vi "InfoRead4.vi"(4 "data info template":refnum<vi>, 5 "source path":string) -> (2 "data from *.info.txt":T1)   [LabVIEW 2014]
uses:
  <vilib>/Utility/file.llb/Read From Spreadsheet File (string).vi
panel:
  # "0 - aplly *.info.txt\n1 - Continue and enter the data manually\n2 - Cancel and correct the *.info.txt"
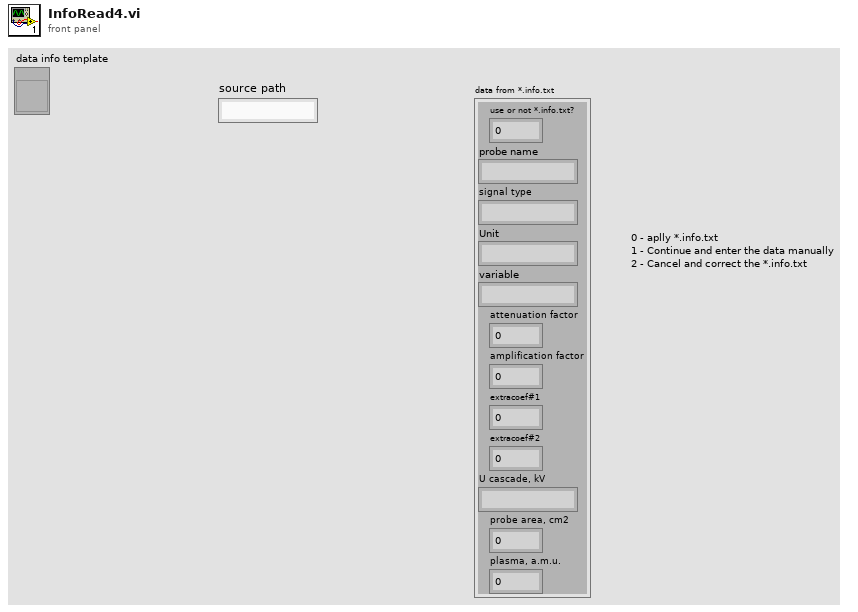
[diagram p1: front panel]
types:
  T1 = cluster{"use or not *.info.txt?":i16, "probe name":string, "signal type":string, "Unit":string, "variable":string, "attenuation factor":dbl, "amplification factor":dbl, "extracoef#1":dbl, "extracoef#2":dbl, "U cascade, kV":string, "probe area, cm2":dbl, "plasma, a.m.u.":dbl}
  T2 = cluster{"data path":string, "ADCintercadr_s":dbl, "data info":cluster{"use or not *.info.txt?":i16, "probe name":string, "signal type":string, "Unit":string, "variable":string, "attenuation factor":dbl, "amplification factor":dbl, "extracoef#1":dbl, "extracoef#2":dbl, "U cascade, kV":string, "probe area, cm2":dbl, "plasma, a.m.u.":dbl}, "channel_name":string, "channels_in_file":i32}
  T3 = enum16{"Left Button", "Center Button", "Right Button", "Window Close"}
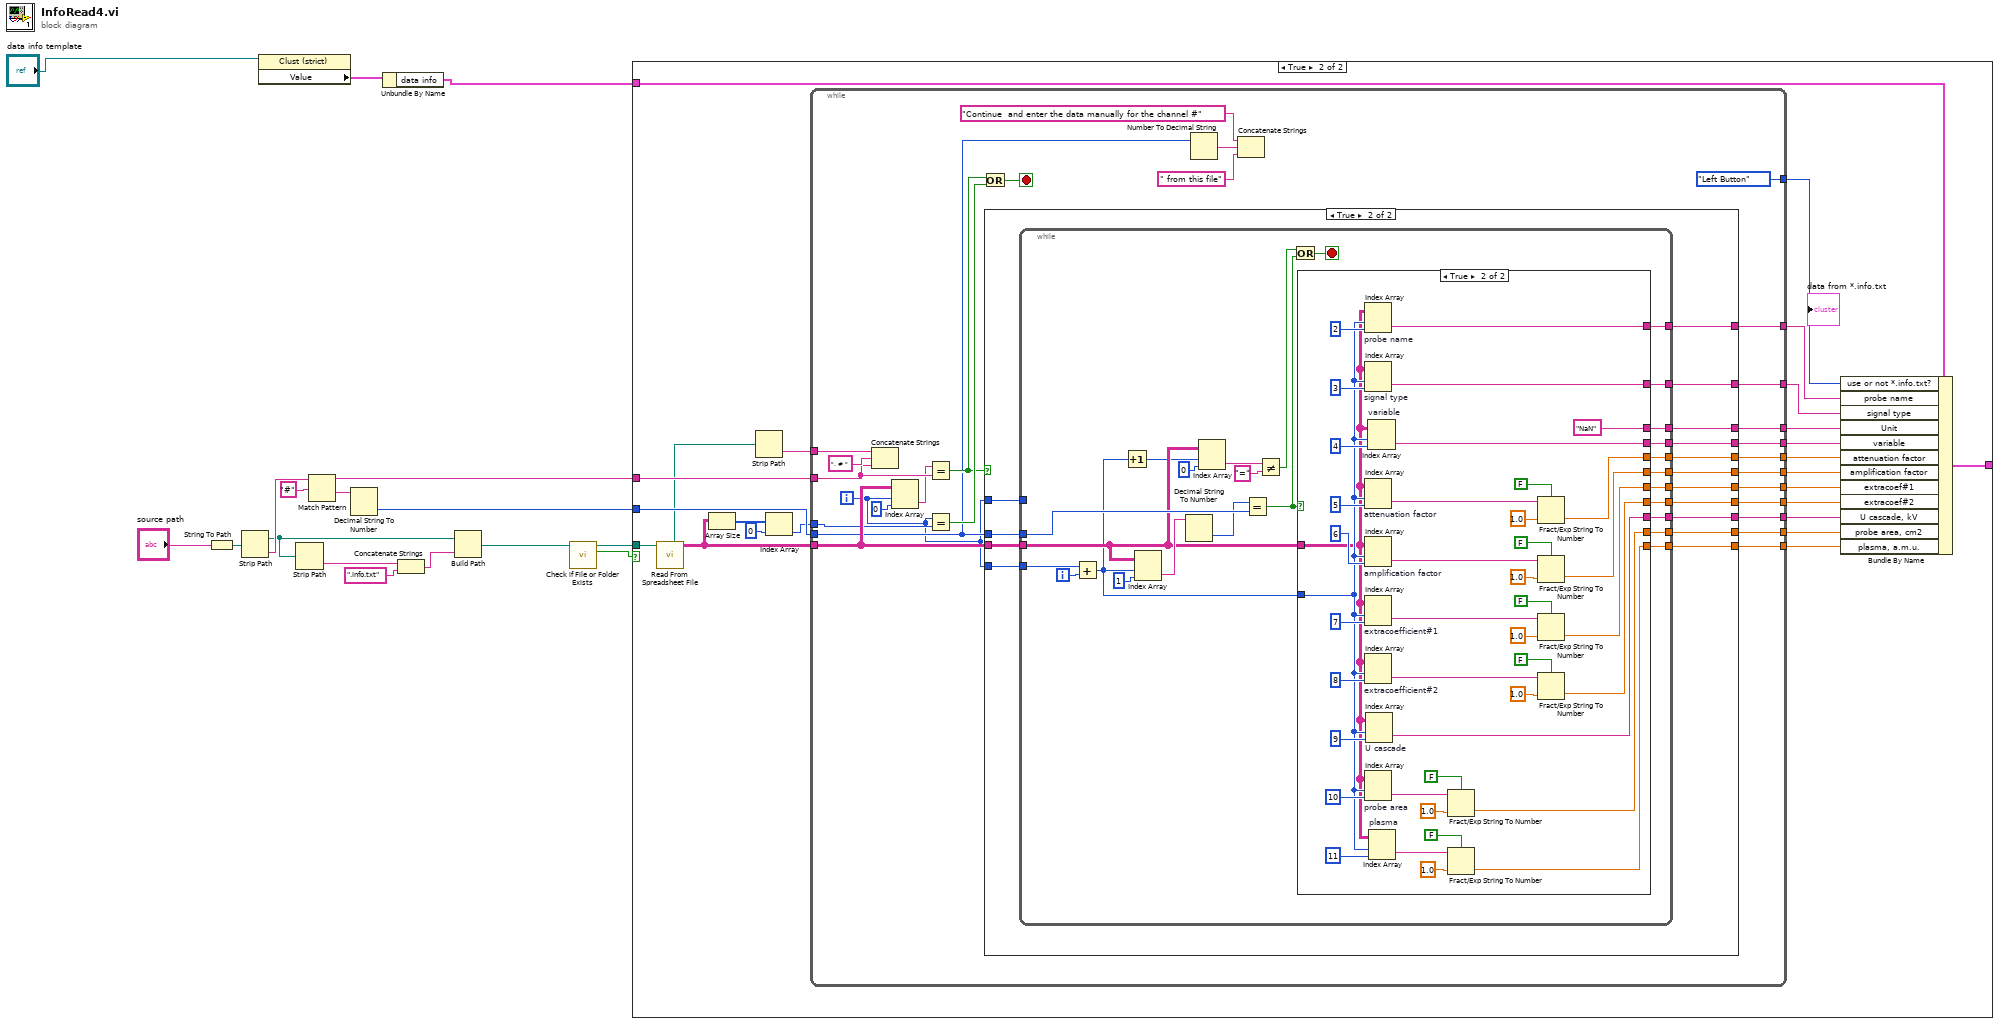
[diagram p0: block diagram]
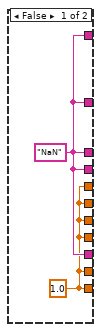
[diagram p3: hidden frame]
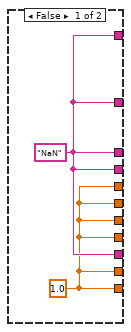
[diagram p4: hidden frame]
diagram:
  n1 = String To Path(string="source path") -> (path=w12:path)
  n2 = Strip Path(path=w12) -> (stripped path=w6:path, name=w16:string)
  n3 = property class="Clust (strict)"(reference="data info template") -> ("Value"=w3:T2)  [unwired: 1 in, 2 out]
  n4 = Strip Path(path=w6) -> (name=w5:string)  [unwired: 1 out]
  n5 = Match Pattern(string=w16, regular expression="#") -> (before substring=w11:string, after substring=w14:string)  [unwired: 1 in, 2 out]
  n6 = Decimal String To Number(string=w14) -> (number=w13:i32)  [unwired: 2 in, 1 out]
  n7 = Unbundle By Name(w3) -> ("data info"=w2:T1)
  n8 = Concatenate Strings(w5, ".info.txt" ("string")) -> (w9:string)
  n9 = Build Path(base path=w6, name or relative path=w9) -> (appended path=w8:path)
  n10 = call <vilib>:"Check if File or Folder Exists.vi"("path"=w8) -> ("file or folder exists?"=w4:bool, "dup path"=w7:path)  [unwired: 8 in, 1 out]
  n11 = case shown="True" w4 {
    tunnel: w13 -> [_ w38]
    tunnel: w11 -> [_ w37]
    tunnel: w7 -> [_ w35]
    tunnel: [w18 w19] -> _
    tunnel: w2 -> [w18 w20]
    frame False {
    }
    frame True {
      n12 = call-poly <vilib>:"Read From Spreadsheet File.vi"("file path (dialog if empty)"=w35) -> ("all rows"=w36:string[][], "new file path (Not A Path if cancelled)"=w34:path)  [unwired: 6 in, 3 out]
      n13 = Array Size(array=w36) -> (size(s)=w40:i32[])
      n14 = Strip Path(path=w34) -> (name=w39:string)  [unwired: 1 out]
      n15 = Index Array(array=w40, index=0) -> (element=w33:i32)
      n16 = while {
        tunnel: w36 -> [w64]
        tunnel: [T3."Left Button" ("Which Button?")] -> w32
        tunnel: w38 -> [w58]
        tunnel: w39 -> [w60]
        tunnel: w37 -> [w57]
        tunnel: w33 -> [w56]
        tunnel: [w55] -> w31
        tunnel: [w54] -> w30
        tunnel: [w53] -> w29
        tunnel: [w52] -> w28
        tunnel: [w51] -> w27
        tunnel: [w50] -> w26
        tunnel: [w49] -> w25
        tunnel: [w48] -> w24
        tunnel: [w47] -> w23
        tunnel: [w46] -> w22
        tunnel: [w45] -> w21
        i -> [w44]
        stop <- w67 stop-if-true
        n17 = Concatenate Strings(w60, ", # " ("string"), w57) -> ()  [unwired: 1 out]
        n18 = Index Array(array=w64, index (row)=w44, index (col)=0 ("disabled index (col)")) -> (element=w43:string)
        n19 = Equal?(x=w43, y=w57) -> (x = y?=w65:bool)
        n20 = Equal?(x=w44, y=w56) -> (x = y?=w66:bool)
        n21 = Or(x=w65, y=w66) -> (x .or. y?=w67:bool)
        n22 = case shown="True" w65 {
          tunnel: w64 -> [_ w72]
          tunnel: w58 -> [_ w85]
          tunnel: w44 -> [_ w84]
          tunnel: [w70 w82] -> w55
          tunnel: [w70 w81] -> w54
          tunnel: [w70 w83] -> w53
          tunnel: [w70 w80] -> w52
          tunnel: [w70 w75] -> w51
          tunnel: [w69 w79] -> w50
          tunnel: [w69 w78] -> w49
          tunnel: [w69 w77] -> w48
          tunnel: [w69 w76] -> w47
          tunnel: [w69 w74] -> w46
          tunnel: [w69 w73] -> w45
          tunnel: w44 -> [_ w71]
          frame False {
            w69 = 1.0
            w70 = "NaN" ("String")
          }
          frame True {
            n23 = while {
              tunnel: w85 -> [w111]
              tunnel: w84 -> [_]
              tunnel: [w110] -> w83
              tunnel: [w109] -> w82
              tunnel: [w108] -> w81
              tunnel: [w107] -> w80
              tunnel: [w106] -> w79
              tunnel: [w105] -> w78
              tunnel: [w104] -> w77
              tunnel: [w103] -> w76
              tunnel: [w102] -> w75
              tunnel: [w101] -> w74
              tunnel: [w100] -> w73
              tunnel: w72 -> [w93]
              tunnel: w71 -> [w97]
              i -> [w96]
              stop <- w88 stop-if-true
              n24 = Add(x=w97, y=w96) -> (x+y=w89:i32)
              n25 = Increment(x=w89) -> (x+1=w90:i32)
              n26 = Index Array(array=w93, index (row)=w89, index (col)=1 ("disabled index (col)")) -> (element=w98:string)
              n27 = Decimal String To Number(string=w98) -> (number=w99:i32)  [unwired: 2 in, 1 out]
              n28 = Index Array(array=w93, index (row)=w90, index (col)=0 ("disabled index (col)")) -> (element=w92:string)
              n29 = Equal?(x=w99, y=w111) -> (x = y?=w86:bool)
              n30 = Not Equal?(x=w92, y="=") -> (x != y?=w87:bool)
              n31 = Or(x=w87, y=w86) -> (x .or. y?=w88:bool)
              n32 = case shown="True" w86 {
                tunnel: [w113 "NaN"] -> w110
                tunnel: [w113 w129] -> w109
                tunnel: [w113 w128] -> w108
                tunnel: [w113 w127] -> w107
                tunnel: [w112 w126] -> w106
                tunnel: [w112 w125] -> w105
                tunnel: [w112 w124] -> w104
                tunnel: w89 -> [_ w122]
                tunnel: [w112 w118] -> w103
                tunnel: [w113 w117] -> w102
                tunnel: [w112 w116] -> w101
                tunnel: [w112 w115] -> w100
                tunnel: w93 -> [_ w114]
                frame False {
                  w112 = 1.0
                  w113 = "NaN"
                }
                frame True {
                  n33 = Index Array "probe name"(array=w114, index (row)=w122, index (col)=2 ("disabled index (col)")) -> (element=w129:string)
                  n34 = Index Array "signal type"(array=w114, index (row)=w122, index (col)=3 ("disabled index (col)")) -> (element=w128:string)
                  n35 = Index Array "attenuation factor"(array=w114, index (row)=w122, index (col)=5 ("disabled index (col)")) -> (element=w139:string)
                  n36 = Index Array "amplification factor"(array=w114, index (row)=w122, index (col)=6 ("disabled index (col)")) -> (element=w140:string)
                  n37 = Index Array "extracoefficient#1"(array=w114, index (row)=w122, index (col)=7 ("disabled index (col)")) -> (element=w147:string)
                  n38 = Index Array "extracoefficient#2"(array=w114, index (row)=w122, index (col)=8 ("disabled index (col)")) -> (element=w119:string)
                  n39 = Index Array "probe area"(array=w114, index (row)=w122, index (col)=10 ("disabled index (col)")) -> (element=w135:string)
                  n40 = Index Array "U cascade"(array=w114, index (row)=w122, index (col)=9 ("disabled index (col)")) -> (element=w117:string)
                  n41 = Index Array "variable"(array=w114, index (row)=w122, index (col)=4 ("disabled index (col)")) -> (element=w127:string)
                  n42 = Index Array "plasma"(array=w114, index (row)=w122, index (col)=11 ("disabled index (col)")) -> (element=w131:string)
                  n43 = Fract/Exp String To Number(use system decimal point (T)=FALSE, string=w135, default (0 dbl)=1.0 ("default (0 DBL)")) -> (number=w116:dbl)  [unwired: 1 in, 1 out]
                  n44 = Fract/Exp String To Number(use system decimal point (T)=FALSE, string=w131, default (0 dbl)=1.0 ("default (0 DBL)")) -> (number=w115:dbl)  [unwired: 1 in, 1 out]
                  n45 = Fract/Exp String To Number(use system decimal point (T)=FALSE, string=w139, default (0 dbl)=1.0 ("default (0 DBL)")) -> (number=w126:dbl)  [unwired: 1 in, 1 out]
                  n46 = Fract/Exp String To Number(use system decimal point (T)=FALSE, string=w140, default (0 dbl)=1.0 ("default (0 DBL)")) -> (number=w125:dbl)  [unwired: 1 in, 1 out]
                  n47 = Fract/Exp String To Number(use system decimal point (T)=FALSE, string=w147, default (0 dbl)=1.0 ("default (0 DBL)")) -> (number=w124:dbl)  [unwired: 1 in, 1 out]
                  n48 = Fract/Exp String To Number(use system decimal point (T)=FALSE, string=w119, default (0 dbl)=1.0 ("default (0 DBL)")) -> (number=w118:dbl)  [unwired: 1 in, 1 out]
                }
              }
            }
          }
        }
        n49 = Number To Decimal String(number=w58) -> (decimal integer string=w62:string)  [unwired: 1 in]
        n50 = Concatenate Strings("Continue  and enter the data manually for the channel #" ("Left Button Text (\"Yes\")"), w62, " from this file" ("string")) -> ()  [unwired: 1 out]
      }
      n51 = Bundle By Name(cluster=w20, "use or not *.info.txt?"=w32, "probe name"=w31, "signal type"=w30, "Unit"=w29, "variable"=w28, "attenuation factor"=w26, "amplification factor"=w25, "extracoef#1"=w24, "extracoef#2"=w23, "U cascade, kV"=w27, "probe area, cm2"=w22, "plasma, a.m.u."=w21) -> (w19:T1)
    }
  }
